vi "Unscale Data.vi"(8 "error in (no error)":errorcluster, 9 "Scaling Info":T1, 10 "Scaled Value":dbl) -> (0 "error out":errorcluster, 2 "Raw Value":u64 format="%016x")   [LabVIEW 2020, in "BCI-1553 API.lvlib"]
doc: "Converts from a double value to a raw U64 representation. The value stored in the U64 depends entirely on the contents of the Scaling Info cluster. Endianness is currently unused."
uses:
  BCI-1553 API.lvlib
  TypeDefs/Scaling Information.ctl
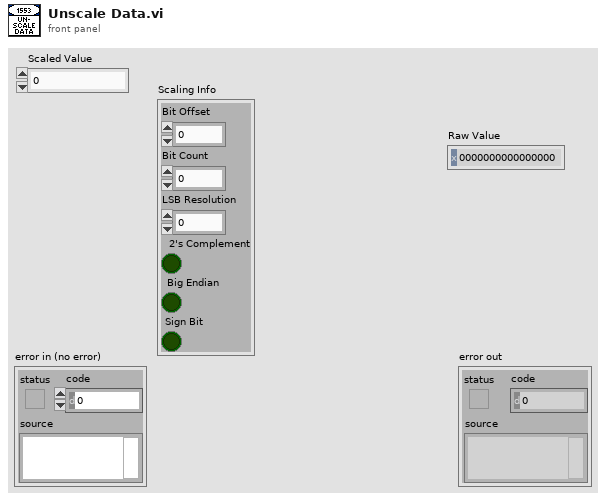
[diagram p1: front panel]
types:
  T1 = typedef "BCI-1553 API.lvlib/Scaling Information.ctl" = cluster{"Bit Offset":i32, "Bit Count":i32, "LSB Resolution":dbl, "2's Complement":bool, "Big Endian":bool, "Sign Bit":bool}
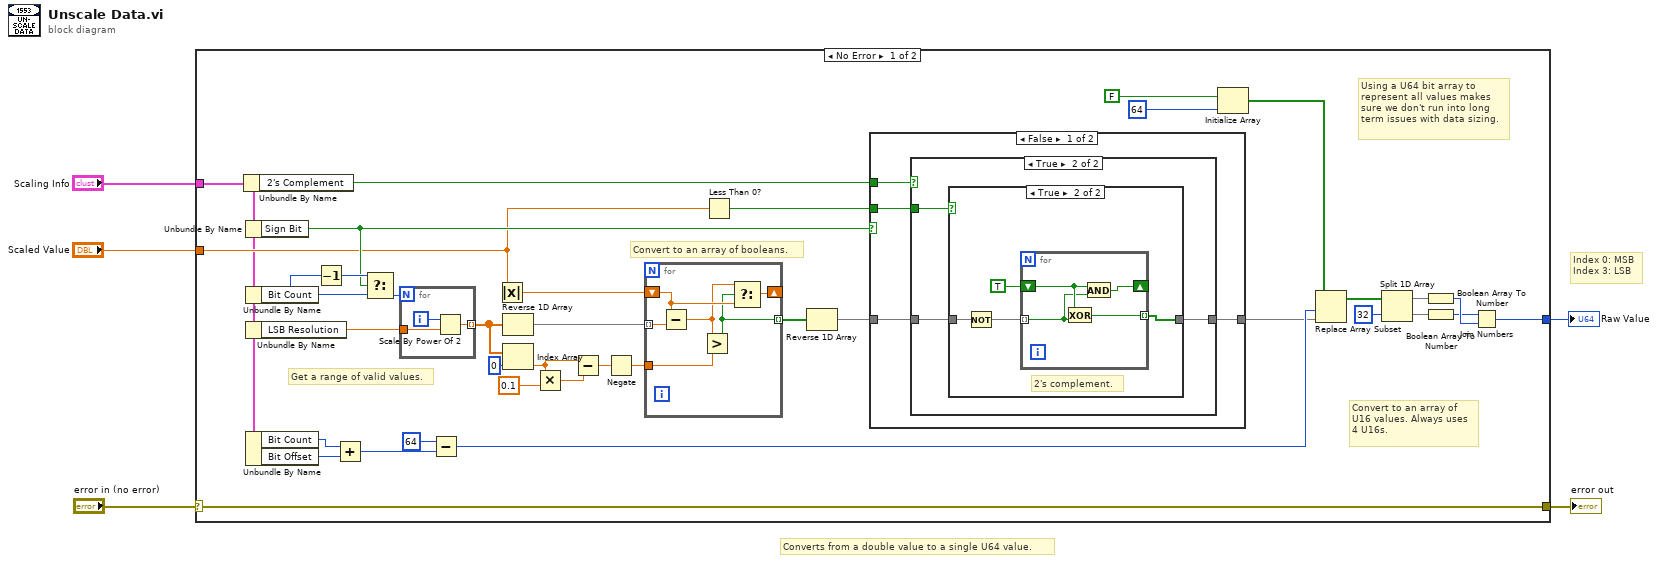
[diagram p0: block diagram]
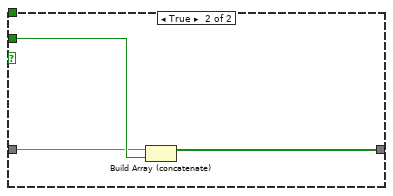
[diagram p4: hidden frame]
diagram:
  # "Index 0: MSB\nIndex 3: LSB"
  # "Converts from a double value to a single U64 value."
  n1 = case shown="No Error" "error in (no error)" {
    selector: "error in (no error)" -> [w42 w72]
    tunnel: [w42 w72] -> w4
    tunnel: "Scaling Info" -> [w9 _]
    tunnel: "Scaled Value" -> [w11 _]
    tunnel: [w25 _] -> w1
    frame No Error {
      # "Using a U64 bit array to\nrepresent all values makes\nsure we don't run into long\nterm issues with data sizing."
      # "Convert to an array of\nU16 values. Always uses\n4 U16s."
      # "Convert to an array of booleans."
      # "Get a range of valid values."
      n2 = Unbundle By Name(w9) -> ("2's Complement"=w8:bool)
      n3 = Unbundle By Name(w9) -> ("Sign Bit"=w12:bool)
      n4 = Unbundle By Name(w9) -> ("Bit Count"=w13:i32)
      n5 = Unbundle By Name(w9) -> ("LSB Resolution"=w41:dbl)
      n6 = Unbundle By Name(w9) -> ("Bit Count"=w24:i32, "Bit Offset"=w23:i32)
      n7 = Decrement(x=w13) -> (x-1=w15:i32)
      n8 = Add(x=w24, y=w23) -> (x+y=w30:i32)
      n9 = Select(t=w15, s=w12, f=w13) -> (s? t:f=w14:i32)
      n10 = for {
        N: w14 -> [_]
        tunnel: w41 -> [w71]
        tunnel: [w69] -> w22 mode=indexing
        i -> [w70]
        n11 = Scale By Power Of 2(n=w70, x=w71) -> (x*2^n=w69:dbl)
      }
      n12 = Subtract(x=64 ("dimension size"), y=w30) -> (x-y=w29:i32)
      n13 = Absolute Value(x=w11) -> (abs(x)=w39:dbl)
      n14 = Reverse 1D Array(array=w22) -> (reversed array=w40:dbl[])
      n15 = Index Array(array=w22, index=0) -> (element=w18:dbl)
      n16 = Multiply(x=w18, y=0.1) -> (x*y=w17:dbl)
      n17 = Subtract(x=w18, y=w17) -> (x-y=w16:dbl)
      n18 = Negate(x=w16) -> (-x=w20:dbl)
      n19 = for {
        tunnel: w40 -> [w67] mode=indexing
        shift-right: [w66] -> _
        shift-left: w39 -> [w68]
        tunnel: [w65] -> w6 mode=indexing
        tunnel: w20 -> [w63]
        n20 = Subtract(x=w68, y=w67) -> (x-y=w64:dbl)
        n21 = Greater?(x=w64, y=w63) -> (0:w65:bool)
        n22 = Select(t=w64, s=w65, f=w68) -> (s? t:f=w66:dbl)
      }
      n23 = Less Than 0?(x=w11) -> (x < 0?=w10:bool)
      n24 = Reverse 1D Array(array=w6) -> (reversed array=w7:bool[])
      n25 = case shown="False" w12 {
        tunnel: w7 -> [w46 w60]
        tunnel: [w45 w62] -> w26
        tunnel: w10 -> [w43 w61]
        tunnel: w8 -> [w44 _]
        frame False {
          n26 = case shown="True" w44 {
            tunnel: w46 -> [w47 w50]
            tunnel: [w47 w49] -> w45
            tunnel: w43 -> [_ w48]
            frame False {
              # "No 2's complement encoding\nrequired."
            }
            frame True {
              n27 = case shown="True" w48 {
                tunnel: w50 -> [w51 w54]
                tunnel: [w51 w52] -> w49
                frame False {
                }
                frame True {
                  # "2's complement."
                  n28 = Not(x=w54) -> (.not. x?=w53:bool[])
                  n29 = for {
                    tunnel: w53 -> [w56] mode=indexing
                    shift-right: [w58] -> _
                    shift-left: TRUE -> [w59]
                    tunnel: [w57] -> w52 mode=indexing
                    n30 = Exclusive Or(1:w56, 2:w59) -> (0:w57:bool)
                    n31 = And(x=w59, y=w56) -> (x .and. y?=w58:bool)
                  }
                }
              }
            }
          }
        }
        frame True {
          n32 = Build Array (concatenate)(w60, w61) -> (w62:bool[])
        }
      }
      n33 = Initialize Array(FALSE, 64 ("dimension size")) -> (w32:bool[])
      n34 = Replace Array Subset(array=w32, new element=w26, index=w29) -> (w36:bool[])
      n35 = Split 1D Array(array=w36, index=32) -> (first subarray=w33:bool[], second subarray=w34:bool[])
      n36 = Boolean Array To Number(Boolean array=w33) -> (number=w28:u32)
      n37 = Boolean Array To Number(Boolean array=w34) -> (number=w27:u32)
      n38 = Join Numbers(hi=w27, lo=w28) -> ((hi.lo)=w25:u64)
    }
    frame Error {
    }
  }
  "error out" <- w4
  "Raw Value" <- w1
